vi "bats.parser.test.Time.Twice.vi"(10 "Expected OrderBook.Command[]":T2[](array[typedef])=[{"type"=enum."Time", "side"=0, "orderId "=0, "quantity"=0, "symbol"=0, "price"=0, "executed.qty"=0, "canceled.qty"=0, "remaining.qty"=0, "seconds"=447000, "nanoseconds"=0, "Add"=FALSE, "Edit"=FALSE, "Remove"=FALSE}, {"type"=enum."Time", "side"=0, "orderId "=0, "quantity"=0, "symbol"=0, "price"=0, "executed.qty"=0, "canceled.qty"=0, "remaining.qty"=0, "seconds"=448000, "nanoseconds"=0, "Add"=FALSE, "Edit"=FALSE, "Remove"=FALSE}] {"symbol" format="%.0x"; "orderId" format="%.0x"; "side" format="%.0x"}) -> ()   [LabVIEW 2020]
uses:
  fpga/common/orderbook.command.type.ctl
  fpga/common/orderbook.command.ctl
  pitch/Time/Time.Parameters.ctl
  pitch/Time/Time.lvclass
panel:
  in  "Time.Parameters.2":T1={"Time"=448000}
  in  "Time.Parameters.1":T1={"Time"=447000}
  out "Passed":bool
  out "OrderBook.Command[]":T2[](array[typedef]) {"symbol" format="%.0x"; "orderId" format="%.0x"; "side" format="%.0x"}
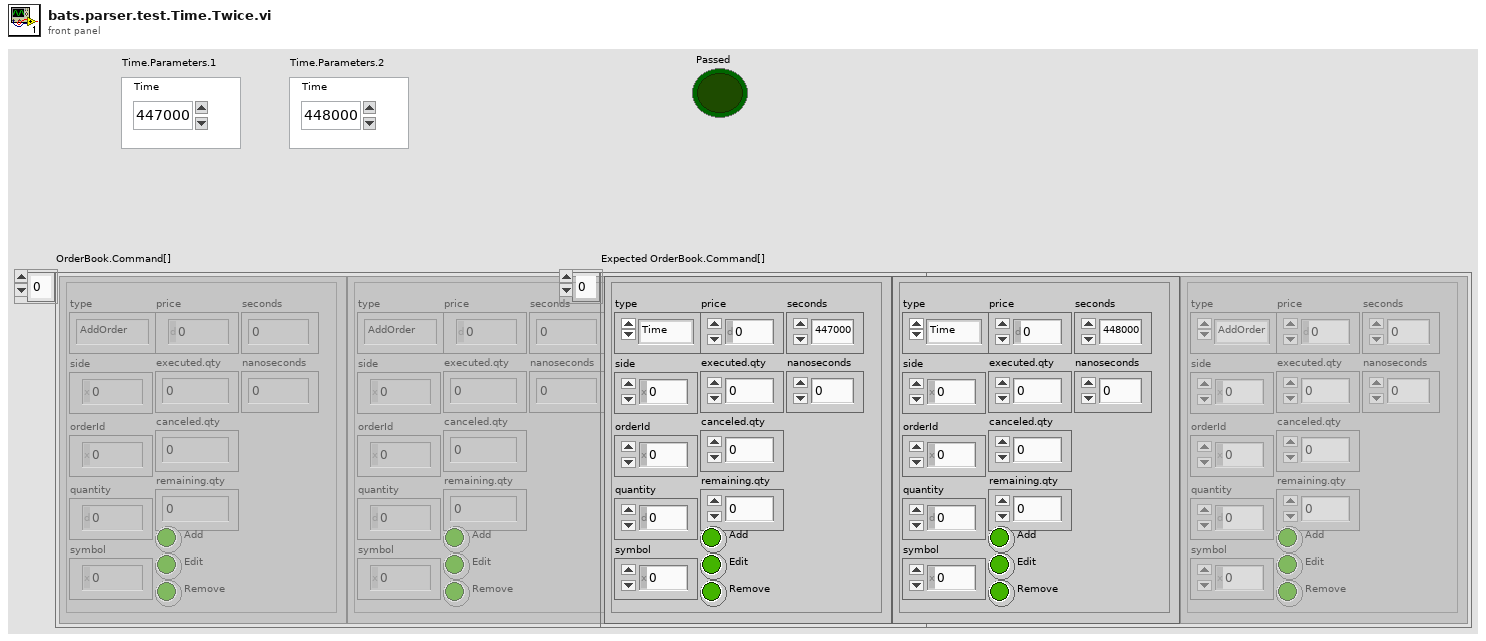
[diagram p1: front panel]
types:
  T1 = typedef "Time.lvclass/Time.Parameters.ctl" = cluster{"Time":u32}
  T2 = typedef "orderbook.command.ctl" = cluster{"type":T3, "side":u8, "orderId ":u64, "quantity":u32, "symbol":u64, "price":u64, "executed.qty":u32, "canceled.qty":u32, "remaining.qty":u32, "seconds":u64, "nanoseconds":u64, "Add":bool, "Edit":bool, "Remove":bool}
  T3 = typedef "orderbook.command.type.ctl" = enum8{"Time", "AddOrder", "OrderExecuted", "OrderExecutedAtPrice", "ReduceSize", "ModifyOrder", "DeleteOrder", "Get.Everything", "Get.All.Orders", "Get.Top"}
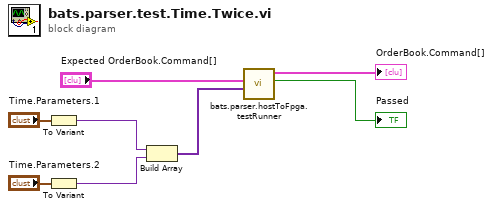
[diagram p0: block diagram]
diagram:
  n1 = To Variant(anything="Time.Parameters.1") -> (Variant=w5:variant)
  n2 = To Variant(anything="Time.Parameters.2") -> (Variant=w4:variant)
  n3 = Build Array(w5, w4) -> (w3:variant[])
  n4 = call "bats.parser.hostToFpga.testRunner.vi"("Test.Messages"=w3, "Expected OrderBook.Command[]"="Expected OrderBook.Command[]") -> ("Passed"=→"Passed":bool, "OrderBook.Command[]"=→"OrderBook.Command[]":T2[])  [unwired: 6 in, 2 out]
